vi "getStrain.vi"(6 "Channel":i32=1 min=1 max=2, 8 "error in (no error)":errorcluster, 11 "Inst.RP100 in":refnum<class "Inst.RP100.lvclass">) -> (0 "error out":errorcluster, 2 "Strain (Ch1) (V)":dbl, 3 "Inst.RP100 out":refnum<class "Inst.RP100.lvclass">)   [LabVIEW 2019, in "Inst.RP100.lvclass"]
uses:
  Inst.RP100.lvclass
  <userlib>/LevyLab/Instrument Framework/Instrument Types/Strain/Instrument.Strain.lvclass
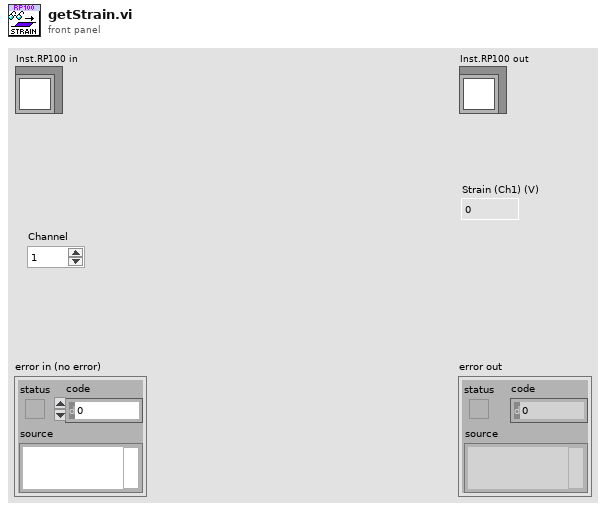
[diagram p1: front panel]
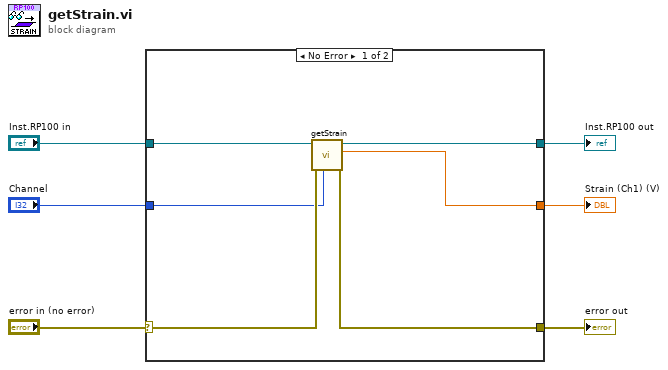
[diagram p0: block diagram]
diagram:
  n1 = case shown="No Error" "error in (no error)" {
    selector: "error in (no error)" -> [w9 w14]
    tunnel: [w8 w14] -> w5
    tunnel: "Inst.RP100 in" -> [w12 w13]
    tunnel: [w10 w13] -> w3
    tunnel: [w11 _] -> w2
    tunnel: "Channel" -> [w7 _]
    frame No Error {
      n2 = call-parent "getStrain.vi"("Channel"=w7, "error in (no error)"=w9, "Instrument.Strain in"=w12) -> ("error out"=w8:errorcluster, "Strain (V)"=w11:dbl, "Instrument.Strain out"=w10:refnum<class "Inst.RP100.lvclass">)  [unwired: 6 in]
    }
    frame Error {
    }
  }
  "error out" <- w5
  "Inst.RP100 out" <- w3
  "Strain (Ch1) (V)" <- w2
